vi "Turn Robot.vi"(2 "Turn Angle":dbl, 3 "RobotDriveDevRef":T1={"DevStatus"={"status"=FALSE, "code"=0, "source"=""}, "Motors[]"=[], "Square Inputs"=FALSE, "Max Output"=1.0}) -> (1 "RobotDriveDevRef Out":T1={"DevStatus"={"status"=FALSE, "code"=0, "source"=""}, "Motors[]"=[], "Square Inputs"=FALSE, "Max Output"=1.0})   [LabVIEW 2016]
uses:
  <vilib>/Rock Robotics/WPI/RobotDrive/WPI_RobotDriveDevRef.ctl
  <vilib>/Rock Robotics/WPI/MotorControl/WPI_MotorControlDeviceRef.ctl
  <vilib>/Rock Robotics/WPI/MotorControl/WPI_MotorControlType.ctl
  <vilib>/Rock Robotics/SystemInterfaces/DIO/FPGA_DIOPWMChannel.ctl
  <vilib>/Rock Robotics/WPI/PWM/WPI_PWMDeadband.ctl
  Robot Global Data.vi
  <vilib>/Rock Robotics/WPI/RobotDrive/WPI_RobotDriveArcadeDrive_Standard(NoSaturation).vi
  <vilib>/Rock Robotics/Network Tables/NT Write Numeric Array.vi
panel:
  out "Iteration":i32
  out "Set Point":dbl
  out "Current Gyro Value":dbl
  out "Gyro Rate":dbl
  out "Centered Time":i32(graph)
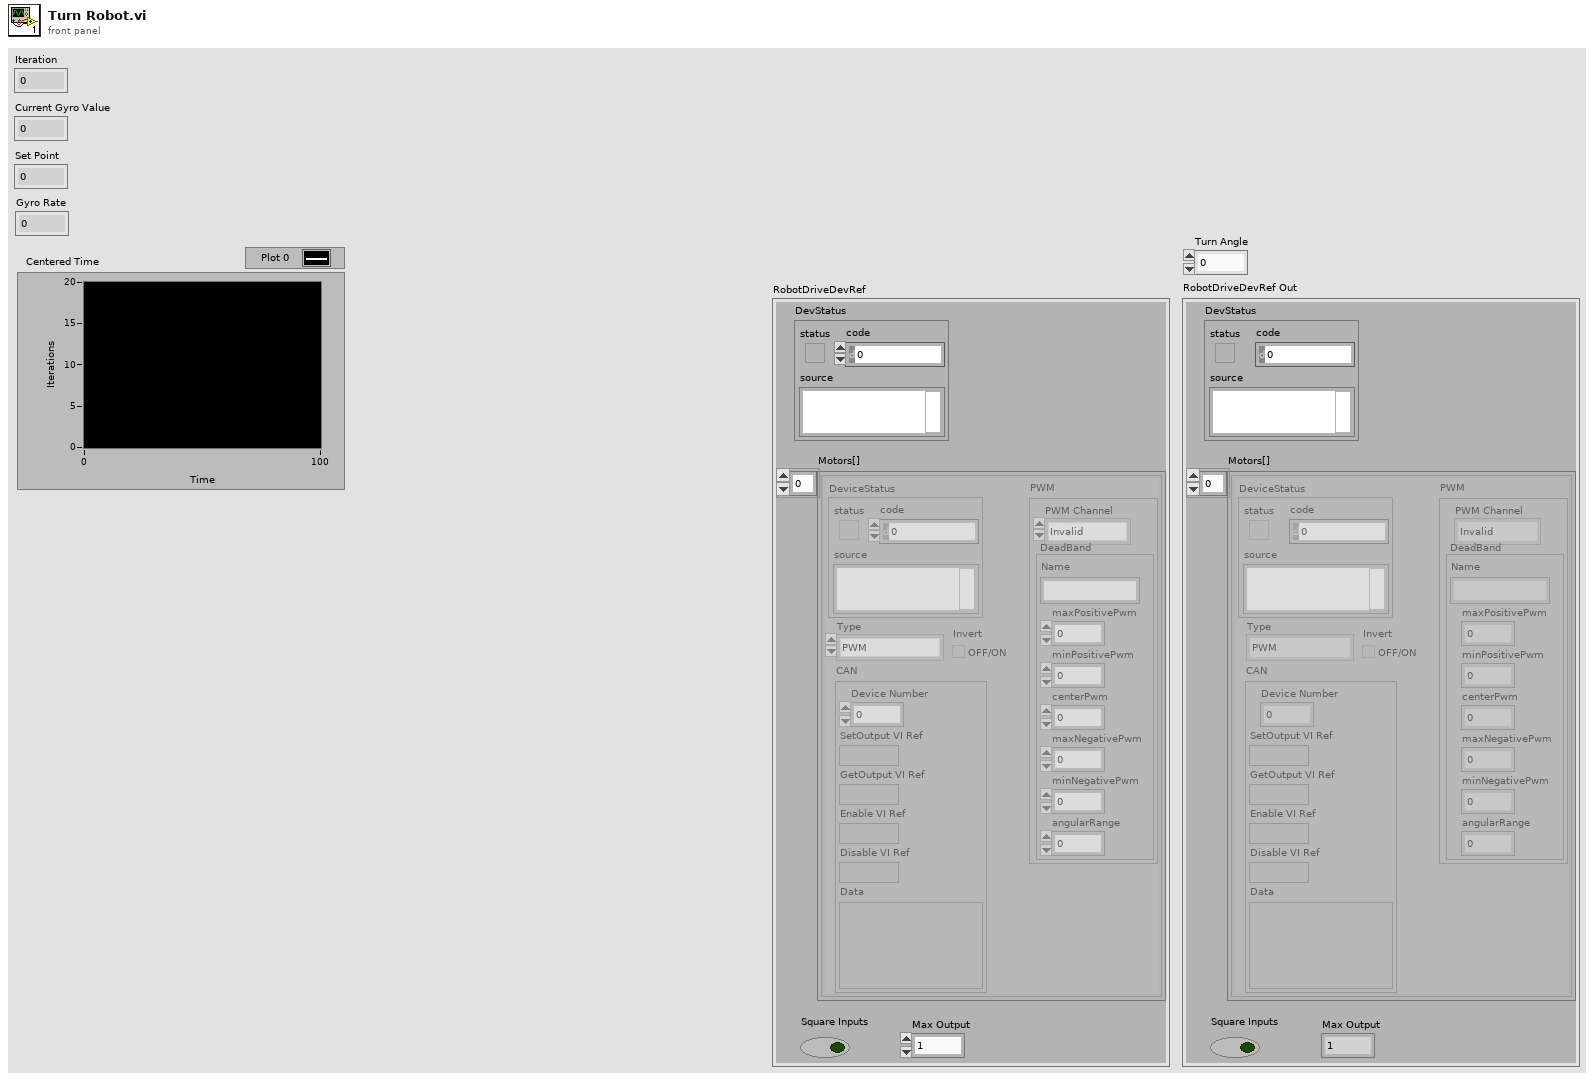
[diagram p1: front panel]
types:
  T1 = typedef "WPI_RobotDriveDevRef.ctl" = cluster{"DevStatus":errorcluster, "Motors[]":T2[], "Square Inputs":bool, "Max Output":dbl}
  T2 = typedef "WPI_MotorControlDeviceRef.ctl" = cluster{"DeviceStatus":errorcluster, "Type":T3, "PWM":cluster{"PWM Channel":T4, "DeadBand":T5}, "CAN":cluster{"Device Number":u8, "SetOutput VI Ref":variant, "GetOutput VI Ref":variant, "Enable VI Ref":variant, "Disable VI Ref":variant, "Data":variant}, "Invert":bool}
  T3 = typedef "WPI_MotorControlType.ctl" = enum16{"PWM", "CAN"}
  T4 = typedef "FPGA_DIOPWMChannel.ctl" = enum8{"PWM 0", "PWM 1", "PWM 2", "PWM 3", "PWM 4", "PWM 5", "PWM 6", "PWM 7", "PWM 8", "PWM 9", "PWM MXP 0", "PWM MXP 1", "PWM MXP 2", "PWM MXP 3", "PWM MXP 4", "PWM MXP 5", "PWM MXP 6", "PWM MXP 7", "PWM MXP 8", "PWM MXP 9", "Invalid"}
  T5 = typedef "WPI_PWMDeadband.ctl" = cluster{"Name":string, "maxPositivePwm":i32, "minPositivePwm":i32, "centerPwm":i32, "maxNegativePwm":i32, "minNegativePwm":i32, "angularRange":u16}
  T6 = cluster{"X Angle":dbl, "Y Angle":dbl, "Z Angle":dbl}
  T7 = typedef "WPI_GyroDevRef.ctl" = cluster{"DevStatus":errorcluster, "Analog Channel":T8, "Offset":dbl, "Gain (VoltsPerDegree/Second)":dbl, "Gyro Type":enum16{"Analog", "XRS450"}, "Handle":i32, "SPI Bus":T9, "Device Found":bool, "Sample Rate":dbl, "Calibrate On Open":bool}
  T8 = typedef "FPGA_AIChannel.ctl" = enum8{"AI 0", "AI 1", "AI 2", "AI 3", "AI MXP 0", "AI MXP 1", "AI MXP 2", "AI MXP 3", "Invalid"}
  T9 = typedef "spi_bus.ctl" = enum16{"SPI On-Board, CS0", "SPI On-Board, CS1", "SPI On-Board, CS2", "SPI On-Board, CS3", "SPI MXP", "Invalid"}
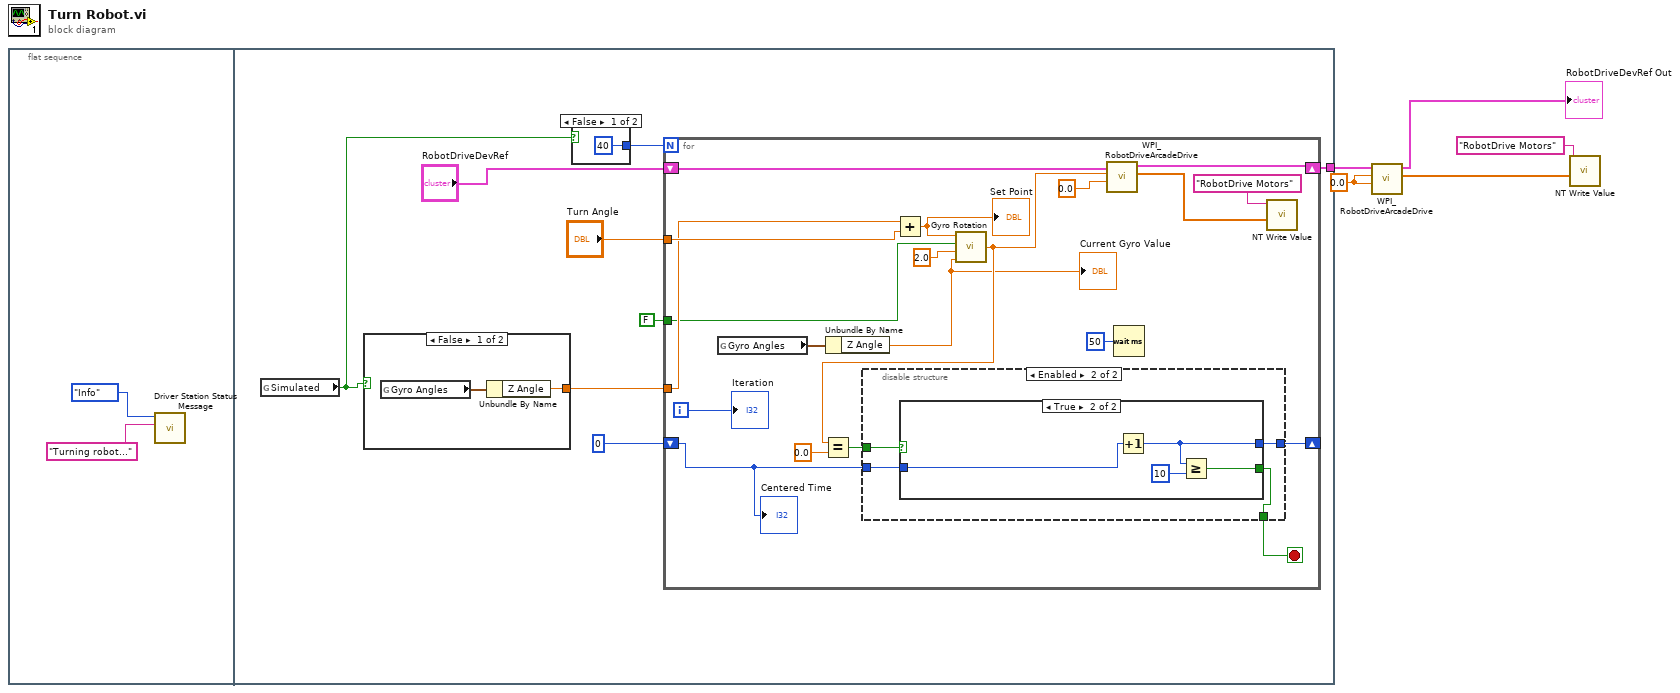
[diagram p0: block diagram]
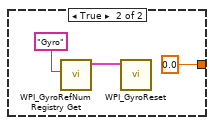
[diagram p2: hidden frame]
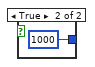
[diagram p3: hidden frame]
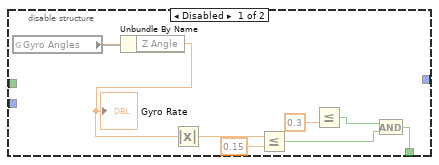
[diagram p4: hidden frame]
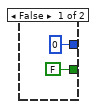
[diagram p5: hidden frame]
diagram:
  w3 = 0.0
  n1 = flat-sequence {
    tunnel: [w13] -> w2
    frame #0 {
      n2 = call "Driver Station Status Message.vi"("Message"="Turning robot...", "Message Type"=enum16{"Error", "Warning", "Info"}."Info") -> ()  [unwired: 10 in]
    }
    frame #1 {
      n3 = global read "Robot Global Data.vi" "Simulated"() -> (w9:bool)
      n4 = case shown="False" w9 {
        tunnel: [w16 0.0 ("Gyro Angle")] -> w10
        frame False {
          n5 = global read "Robot Global Data.vi" "Gyro Angles"() -> (w17:T6)
          n6 = Unbundle By Name(w17) -> ("Z Angle"=w16:dbl)
        }
        frame True {
          n7 = call <vilib>:"WPI_GyroRefNum Registry Get.vi"("refnum name"="Gyro") -> ("GyroDevRef"=w19:T7)  [unwired: 9 in, 1 out]
          n8 = call <vilib>:"WPI_GyroReset.vi"("GyroDevRef"=w19) -> ()  [unwired: 9 in, 2 out]
        }
      }
      n9 = case shown="False" w9 {
        tunnel: [40 1000] -> w15
        frame False {
        }
        frame True {
        }
      }
      n10 = for {
        N: w15 -> [_]
        tunnel: "Turn Angle" -> [w38]
        tunnel: w10 -> [w37]
        tunnel: FALSE -> [w25]
        shift-right: [w32] -> _
        shift-left: 0 -> [w31]
        shift-right: [w30] -> w13
        shift-left: "RobotDriveDevRef" -> [w41]
        i -> [w39]
        stop <- w28 stop-if-true
        n11 = global read "Robot Global Data.vi" "Gyro Angles"() -> (w29:T6)
        n12 = Unbundle By Name(w29) -> ("Z Angle"=w23:dbl)
        "Current Gyro Value" <- w23
        n13 = Add(x=w37, y=w38) -> (x+y=w26:dbl)
        "Set Point" <- w26
        n14 = call "Gyro Rotation.vi"("Current Value"=w23, "Deadband"=2.0, "Invert Rotation"=w25, "Set Point"=w26) -> ("Rotation"=w27:dbl)
        n15 = Equal?(x=w27, y=0.0) -> (x = y?=w33:bool)
        n16 = disable-structure shown="Enabled" {
          disable-tunnel: [w46 w52] -> w28
          disable-tunnel: w33 -> [_ w55]
          disable-tunnel: [_ w54] -> w32
          disable-tunnel: w31 -> [_ w53]
          frame Disabled {
            n17 = global read "Robot Global Data.vi" "Gyro Angles"() -> (w44:T6)
            n18 = Unbundle By Name(w44) -> ("Z Angle"=w43:dbl)
            "Gyro Rate" <- w43
            n19 = Absolute Value(x=w43) -> (abs(x)=w50:dbl)
            n20 = Less Or Equal?(x=w50, y=0.15) -> (x <= y?=w48:bool)
            n21 = Less Or Equal?(y=0.3) -> (x=w45:dbl, x <= y?=w47:bool)
            n22 = And(x=w47, y=w48) -> (x .and. y?=w46:bool)
          }
          frame Enabled {
            n23 = case shown="True" w55 {
              tunnel: [0 w60] -> w54
              tunnel: w53 -> [_ w61]
              tunnel: [FALSE w58] -> w52
              frame False {
              }
              frame True {
                n24 = Increment(x=w61) -> (x+1=w60:i32)
                n25 = Greater Or Equal?(x=w60, y=10) -> (x >= y?=w58:bool)
              }
            }
          }
        }
        n26 = call-poly <vilib>:"WPI_RobotDriveArcadeDrive.vi"("Y axis value"=0.0, "X axis value"=w27, "RobotDriveDevRef"=w41) -> ("Motor Values"=w35:dbl[], "RobotDriveDevRef"=w30:T1)  [unwired: 6 in, 1 out]
        n27 = Wait (ms)(milliseconds to wait=u32 50) -> ()  [unwired: 1 out]
        n28 = call-poly <vilib>:"NT Write Value.vi"("Numeric Array"=w35, "Name"="RobotDrive Motors") -> ()  [unwired: 9 in, 1 out]
        "Iteration" <- w39
        "Centered Time" <- w31
      }
    }
  }
  n29 = call-poly <vilib>:"WPI_RobotDriveArcadeDrive.vi"("Y axis value"=w3, "X axis value"=w3, "RobotDriveDevRef"=w2) -> ("Motor Values"=w5:dbl[], "RobotDriveDevRef"=→"RobotDriveDevRef Out":T1)  [unwired: 6 in, 1 out]
  n30 = call-poly <vilib>:"NT Write Value.vi"("Numeric Array"=w5, "Name"="RobotDrive Motors") -> ()  [unwired: 9 in, 1 out]
